vi "ArmIncrementXYZ.vi"(9 "AddZ":dbl, 10 "AddY":dbl, 11 "AddX":dbl) -> ()   [LabVIEW 2020]
doc: "Increment X,Y,Z values\n\nInput:\n--AddX--Double--how much to increment X\n--AddY--Double--how much to increment Y\n--AddZ--Double--how much to increment Z"
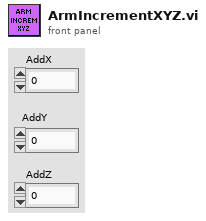
[diagram p1: front panel]
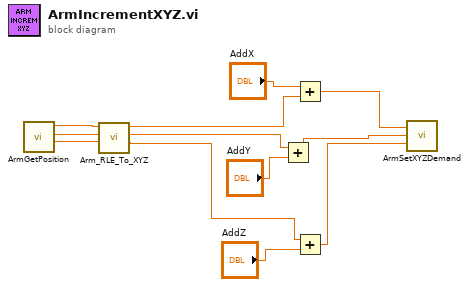
[diagram p0: block diagram]
diagram:
  n1 = call "ArmGetPosition.vi"() -> ("ExtendPostion"=w4:dbl, "LiftPostion"=w5:dbl, "RotatePostion"=w6:dbl)  [unwired: 9 in]
  n2 = call "Arm_RLE_To_XYZ.vi"("Extend"=w4, "Lift"=w5, "Rotate"=w6) -> ("z"=w1:dbl, "y"=w2:dbl, "x"=w3:dbl)  [unwired: 6 in]
  n3 = Add(x=w2, y="AddY") -> (x+y=w8:dbl)
  n4 = Add(x="AddX", y=w3) -> (x+y=w9:dbl)
  n5 = Add(x=w1, y="AddZ") -> (x+y=w7:dbl)
  n6 = call "ArmSetXYZDemand.vi"("SetZ"=w7, "SetY"=w8, "SetX"=w9) -> ()  [unwired: 9 in]
